vi "Render Template.vi"(6 "Locals (None)":map{string, string}(c390), 7 "Folder":path, 8 "error in (no error)":errorcluster, 10 "Template":string, 11 "TemplateService in":refnum<class "TemplateService.lvclass">) -> (0 "error out":errorcluster, 2 "Output":string, 3 "TemplateService out":refnum<class "TemplateService.lvclass">)   [LabVIEW 2020, in "HTTP Server.lvlib" / "TemplateService.lvclass"]
uses:
  TemplateService.lvclass
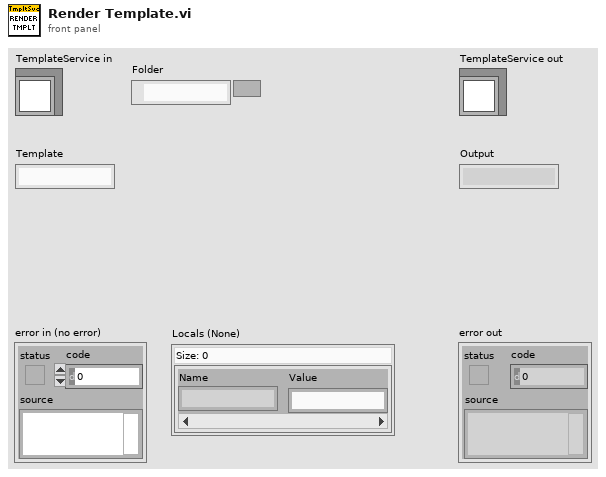
[diagram p1: front panel]
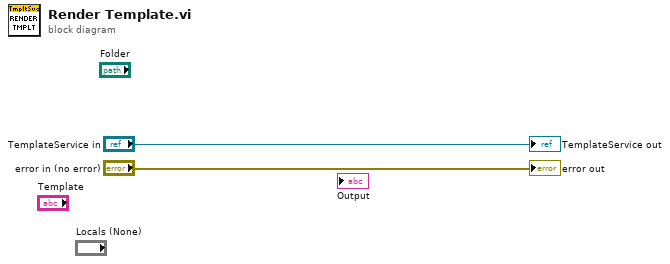
[diagram p0: block diagram]
diagram:
  "error out" <- "error in (no error)"
  "TemplateService out" <- "TemplateService in"
